vi "ConfigurePigeonMP.vi"(8 "Pigeon Talon":T1, 9 "Pigeon":T6 {"Type" items=["CAN"=352321536, "TalonSRX"=33554432]}, 10 "Right Side":T1, 11 "Left Side":T1) -> (1 "Pigeon":T6 {"Type" items=["CAN"=352321536, "TalonSRX"=33554432]}, 2 "Right Side":T1, 3 "Left Side":T1)   [LabVIEW 2018]
uses:
  <vilib>/Rock Robotics/WPI/ThirdParty/Phoenix-LabVIEW/Pigeon IMU/CTRE_PigeonIMU_DeviceRef.ctl
  <vilib>/Rock Robotics/WPI/ThirdParty/Phoenix-LabVIEW/Pigeon IMU/CTRE_PigeonIMU_ConnectionType.ctl
  <vilib>/Rock Robotics/WPI/MotorControl/WPI_MotorControlDeviceRef.ctl
  <vilib>/Rock Robotics/WPI/MotorControl/WPI_MotorControlType.ctl
  <vilib>/Rock Robotics/SystemInterfaces/DIO/FPGA_DIOPWMChannel.ctl
  <vilib>/Rock Robotics/WPI/PWM/WPI_PWMDeadband.ctl
  <vilib>/Rock Robotics/SystemInterfaces/DIO/FPGA_DIOChannel.ctl
  <vilib>/Rock Robotics/WPI/ThirdParty/Phoenix-LabVIEW/Motor Controller/Controls/CTRE_Phoenix_MotorControl_FeedbackDevice.ctl
  <vilib>/Rock Robotics/WPI/ThirdParty/Phoenix-LabVIEW/Motor Controller/Controls/CTRE_Phoenix_MotorControl_RemoteSourceType.ctl
  <vilib>/Rock Robotics/WPI/ThirdParty/Phoenix-LabVIEW/Motor Controller/Controls/CTRE_Phoenix_MotorControl_SensorTermFeedbackDevice_Enhanced.ctl
  <vilib>/Rock Robotics/WPI/ThirdParty/Phoenix-LabVIEW/Motor Controller/Controls/CTRE_Phoenix_MotorControl_StatusFrameEnhanced.ctl
  <vilib>/Rock Robotics/WPI/ThirdParty/Phoenix-LabVIEW/Motor Controller/Controls/CTRE_Phoenix_MotorControl_NeutralMode.ctl
  <vilib>/Rock Robotics/WPI/ThirdParty/Phoenix-LabVIEW/Motor Controller/Controls/CTRE_Phoenix_MotorControl_ControlMode.ctl
  <vilib>/Rock Robotics/WPI/ThirdParty/Phoenix-LabVIEW/Controls/CTRE_Phoenix_Params.ctl
  <vilib>/Rock Robotics/WPI/ThirdParty/Phoenix-LabVIEW/Motor Controller/Controls/CTRE_Phoenix_MotorControl_ControlFrameEnhanced.ctl
  Constants.vi
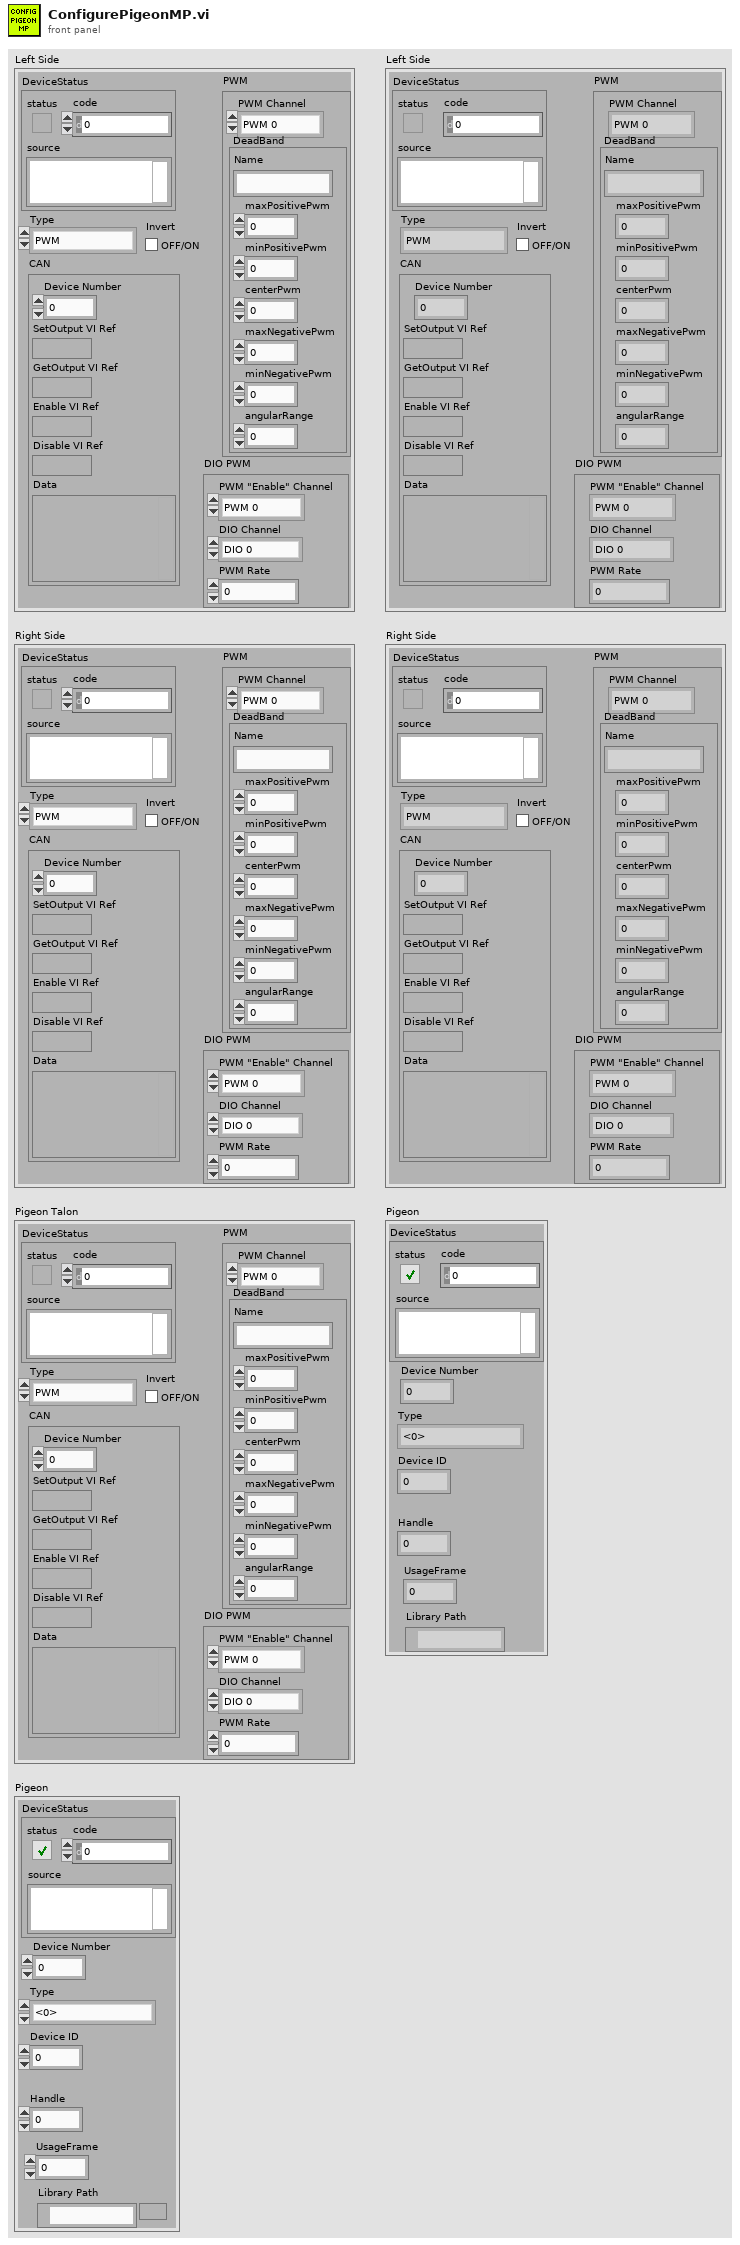
[diagram p1: front panel]
types:
  T1 = typedef "WPI_MotorControlDeviceRef.ctl" = cluster{"DeviceStatus":errorcluster, "Type":T2, "PWM":cluster{"PWM Channel":T3, "DeadBand":T4}, "CAN":cluster{"Device Number":u8, "SetOutput VI Ref":variant, "GetOutput VI Ref":variant, "Enable VI Ref":variant, "Disable VI Ref":variant, "Data":variant}, "Invert":bool, "DIO PWM":cluster{"PWM \"Enable\" Channel":T3, "DIOChannel":T5, "PWM Rate":dbl}}
  T2 = typedef "WPI_MotorControlType.ctl" = enum16{"PWM", "CAN", "DIO PWM"}
  T3 = typedef "FPGA_DIOPWMChannel.ctl" = enum8{"PWM 0", "PWM 1", "PWM 2", "PWM 3", "PWM 4", "PWM 5", "PWM 6", "PWM 7", "PWM 8", "PWM 9", "PWM MXP 0", "PWM MXP 1", "PWM MXP 2", "PWM MXP 3", "PWM MXP 4", "PWM MXP 5", "PWM MXP 6", "PWM MXP 7", "PWM MXP 8", "PWM MXP 9", "Invalid"}
  T4 = typedef "WPI_PWMDeadband.ctl" = cluster{"Name":string, "maxPositivePwm":i32, "minPositivePwm":i32, "centerPwm":i32, "maxNegativePwm":i32, "minNegativePwm":i32, "angularRange":u16}
  T5 = typedef "FPGA_DIOChannel.ctl" = enum8{"DIO 0", "DIO 1", "DIO 2", "DIO 3", "DIO 4", "DIO 5", "DIO 6", "DIO 7", "DIO 8", "DIO 9", "DIO MXP 0", "DIO MXP 1", "DIO MXP 2", "DIO MXP 3", "DIO MXP 4", "DIO MXP 5", "DIO MXP 6", "DIO MXP 7", "DIO MXP 8", "DIO MXP 9", "DIO MXP 10", "DIO MXP 11", "DIO MXP 12", "DIO MXP 13", "DIO MXP 14", "DIO MXP 15", "SPI Port CS1", "SPI Port CS2", "SPI Port CS3", "SPI Port MISO", "SPI Port MOSI", "Invalid"}
  T6 = typedef "CTRE_PigeonIMU_DeviceRef.ctl" = cluster{"DeviceStatus":errorcluster, "Device Number":u8, "Type":T7, "Device ID":u32, "Handle":u64, "UsageFrame":u32, "Library Path":path}
  T7 = typedef "CTRE_PigeonIMU_ConnectionType.ctl" = u32
  T8 = typedef "CTRE_Phoenix_MotorControl_ControlFrameEnhanced.ctl" = u32
  T9 = typedef "CTRE_Phoenix_MotorControl_StatusFrameEnhanced.ctl" = u16
  T10 = typedef "CTRE_Phoenix_Params.ctl" = u16
  T11 = typedef "CTRE_Phoenix_MotorControl_ControlMode.ctl" = u16
  T12 = typedef "CTRE_Phoenix_MotorControl_NeutralMode.ctl" = enum8{"EEPROMSetting", "Override to Coast", "Override to Brake"}
  T13 = typedef "CTRE_Phoenix_MotorControl_FeedbackDevice.ctl" = i8
  T14 = typedef "CTRE_Phoenix_MotorControl_SensorTermFeedbackDevice_Enhanced.ctl" = i8
  T15 = typedef "CTRE_Phoenix_MotorControl_RemoteSourceType.ctl" = enum16{"Off", "Talon SRX Selected Sensor", "Pigeon IMU Yaw", "Pigeon IMU Pitch", "Pigeon IMU Roll", "CANifier Quadrature", "CANifier PWM Input 0", "CANifier PWM Input 1", "CANifier PWM Input 2", "CANifier PWM Input 3", "Gadgeteer Pigeon Yaw", "Gadgeteer Pigeon Pitch", "Gadgeteer Pigeon Roll"}
  T16 = cluster{"kP":dbl, "kI ":dbl, "kD":dbl, "kF":dbl, "I Zone":dbl, "Peak Out":dbl}
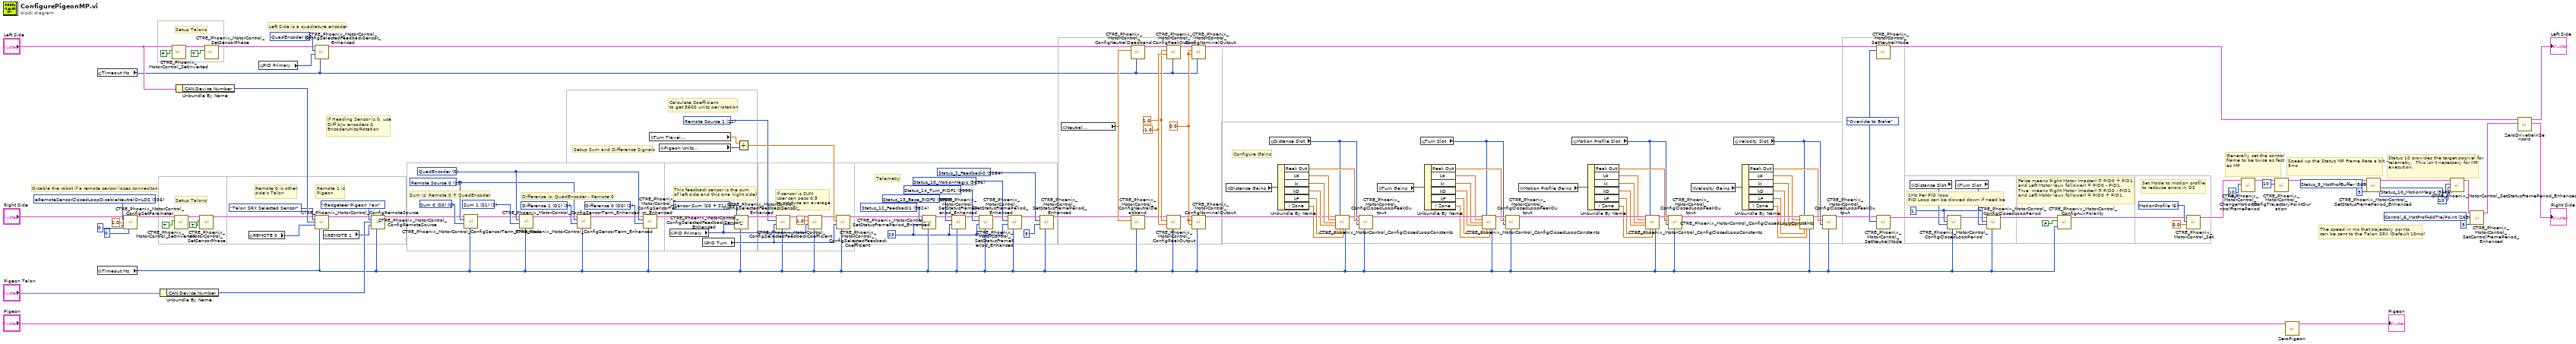
[diagram p0: block diagram]
diagram:
  w6 = T8 262464 items=["Control_3_General"=262272, "Control_4_Advanced"=262336, "Control_5_FeedbackOutputOverride"=262400, "Control_6_MotProfAddTrajPoint"=262464] ("Control Frame")
  w12 = T9 5696 items=["Status_1_General"=5120, "Status_2_Feedback0"=5184, "Status_3_Quadrature"=5248, "Status_4_AinTempVbat"=5312, "Status_6_Misc"=5440, "Status_7_CommStatus"=5504, "Status_8_PulseWidth"=5568, "Status_9_MotProfBuffer"=5632, "Status_10_MotionMagic"=5696, "Status_11_UartGadgeteer"=5760, "Status_12_Feedback1"=5824, "Status_13_Base_PIDF0"=5888, "Status_14_Turn_PIDF1"=5952, "Status_15_FirmwareApiStatus"=6016] ("Status Frame")
  w14 = T9 5632 items=["Status_1_General"=5120, "Status_2_Feedback0"=5184, "Status_3_Quadrature"=5248, "Status_4_AinTempVbat"=5312, "Status_6_Misc"=5440, "Status_7_CommStatus"=5504, "Status_8_PulseWidth"=5568, "Status_9_MotProfBuffer"=5632, "Status_10_MotionMagic"=5696, "Status_11_UartGadgeteer"=5760, "Status_12_Feedback1"=5824, "Status_13_Base_PIDF0"=5888, "Status_14_Turn_PIDF1"=5952, "Status_15_FirmwareApiStatus"=6016] ("Status Frame")
  w20 = T10 336 items=["eOnBoot_BrakeMode"=31, "eQuadFilterEn"=91, "eQuadIdxPolarity"=108, "eClearPositionOnIdx"=100, "eMotionProfileHasUnderrunErr"=119, "eMotionProfileTrajectoryPointDurationMs"=120, "eClearPosOnLimitF"=144, "eClearPosOnLimitR"=145, "eStatusFramePeriod"=300, "eOpenLoopRamp"=301, "eClosedLoopRamp"=302, "eNeutralDeadband"=303, "ePeakPosOutput"=305, "eNominalPosOutput"=306, "ePeakNegOutput"=307, "eNominalNegOutput"=308, "eProfileParamSlot_P"=310, "eProfileParamSlot_I"=311, "eProfileParamSlot_D"=312, "eProfileParamSlot_F"=313, "eProfileParamSlot_IZone"=314, "eProfileParamSlot_AllowableErr"=315, "eProfileParamSlot_MaxIAccum"=316, "eClearPositionOnLimitF"=320, "eClearPositionOnLimitR"=321, "eClearPositionOnQuadIdx"=322, "eSampleVelocityPeriod"=325, "eSampleVelocityWindow"=326, "eFeedbackSensorType"=330, "eSelectedSensorPosition"=331, "eFeedbackNotContinuous"=332, "eRemoteSensorSource"=333, "eRemoteSensorDeviceID"=334, "eSensorTerm"=335, "eRemoteSensorClosedLoopDisableNeutralOnLOS"=336, "eForwardSoftLimitThreshold"=340, "eReverseSoftLimitThreshold"=341, "eForwardSoftLimitEnable"=342, "eReverseSoftLimitEnable"=343, "eNominalBatteryVoltage"=350, "eBatterVoltageFilterSize"=351, "eContinuousCurrentLimitAmps"=360, "eContinuousCurrentLimitMs"=361, "ePeakCurrentLimitAmps"=362, "eClosedLoopIAccum"=370, "eCustomParam"=380, "eStickyFaults"=390, "eAnalogPosition"=400, "eQuadraturePosition"=401, "ePulseWidthPosition"=402, "eMotMag_Accel"=410, "eMotMag_VelCruise"=411, "eLimitSwitchSource"=421, "eLimitSwitchNormClosedAndDis"=422, "eLimitSwitchDisabledNeutralOnLOS"=423, "eLimitSwitchRemoteDevID"=424] ("Parameter")
  w32 = T11 6 items=["PercentOutput"=0, "Position"=1, "Velocity"=2, "Current"=3, "Follower"=5, "MotionProfile"=6, "MotionMagic"=7, "MotionProfileArc"=10, "Disabled"=15] ("Control Mode")
  w140 = 1 ("loopTimeMs")
  w136 = CTRE_Phoenix_MotorControl_NeutralMode."Override to Brake" ("Motor Control Neutral Mode")
  w97 = 0.0 ("Forward Nominal Percent Output")
  w94 = -1.0 ("Reverse Peak Percent Output")
  w93 = 1.0 ("Forward Peak Percent Output")
  w29 = 20 ("periodMs")
  w86 = T9 5184 items=["Status_1_General"=5120, "Status_2_Feedback0"=5184, "Status_3_Quadrature"=5248, "Status_4_AinTempVbat"=5312, "Status_6_Misc"=5440, "Status_7_CommStatus"=5504, "Status_8_PulseWidth"=5568, "Status_9_MotProfBuffer"=5632, "Status_10_MotionMagic"=5696, "Status_11_UartGadgeteer"=5760, "Status_12_Feedback1"=5824, "Status_13_Base_PIDF0"=5888, "Status_14_Turn_PIDF1"=5952, "Status_15_FirmwareApiStatus"=6016] ("Status Frame")
  w85 = T9 5696 items=["Status_1_General"=5120, "Status_2_Feedback0"=5184, "Status_3_Quadrature"=5248, "Status_4_AinTempVbat"=5312, "Status_6_Misc"=5440, "Status_7_CommStatus"=5504, "Status_8_PulseWidth"=5568, "Status_9_MotProfBuffer"=5632, "Status_10_MotionMagic"=5696, "Status_11_UartGadgeteer"=5760, "Status_12_Feedback1"=5824, "Status_13_Base_PIDF0"=5888, "Status_14_Turn_PIDF1"=5952, "Status_15_FirmwareApiStatus"=6016] ("Status Frame")
  w84 = T9 5952 items=["Status_1_General"=5120, "Status_2_Feedback0"=5184, "Status_3_Quadrature"=5248, "Status_4_AinTempVbat"=5312, "Status_6_Misc"=5440, "Status_7_CommStatus"=5504, "Status_8_PulseWidth"=5568, "Status_9_MotProfBuffer"=5632, "Status_10_MotionMagic"=5696, "Status_11_UartGadgeteer"=5760, "Status_12_Feedback1"=5824, "Status_13_Base_PIDF0"=5888, "Status_14_Turn_PIDF1"=5952, "Status_15_FirmwareApiStatus"=6016] ("Status Frame")
  w83 = T9 5888 items=["Status_1_General"=5120, "Status_2_Feedback0"=5184, "Status_3_Quadrature"=5248, "Status_4_AinTempVbat"=5312, "Status_6_Misc"=5440, "Status_7_CommStatus"=5504, "Status_8_PulseWidth"=5568, "Status_9_MotProfBuffer"=5632, "Status_10_MotionMagic"=5696, "Status_11_UartGadgeteer"=5760, "Status_12_Feedback1"=5824, "Status_13_Base_PIDF0"=5888, "Status_14_Turn_PIDF1"=5952, "Status_15_FirmwareApiStatus"=6016] ("Status Frame")
  w82 = T9 5824 items=["Status_1_General"=5120, "Status_2_Feedback0"=5184, "Status_3_Quadrature"=5248, "Status_4_AinTempVbat"=5312, "Status_6_Misc"=5440, "Status_7_CommStatus"=5504, "Status_8_PulseWidth"=5568, "Status_9_MotProfBuffer"=5632, "Status_10_MotionMagic"=5696, "Status_11_UartGadgeteer"=5760, "Status_12_Feedback1"=5824, "Status_13_Base_PIDF0"=5888, "Status_14_Turn_PIDF1"=5952, "Status_15_FirmwareApiStatus"=6016] ("Status Frame")
  w27 = T13 12 items=["None"=-1, "QuadEncoder"=0, "Analog"=2, "Tachometer"=4, "Pulse Width Encoded Position"=8, "Sensor Sum (S0 + S1)"=9, "Sensor Difference (D0 - D1)"=10, "Remote Source 0"=11, "Remote Source 1"=12, "Software Emulated"=15] ("Feedback Device")
  w69 = T13 9 items=["None"=-1, "QuadEncoder"=0, "Analog"=2, "Tachometer"=4, "Pulse Width Encoded Position"=8, "Sensor Sum (S0 + S1)"=9, "Sensor Difference (D0 - D1)"=10, "Remote Source 0"=11, "Remote Source 1"=12, "Software Emulated"=15] ("Feedback Device")
  w67 = u16 2 items=["Sum 0 (S0)", "Sum 1 (S1)", "Difference 0 (D0)", "Difference 1 (D1)"] ("Sensor Term")
  w66 = u16 3 items=["Sum 0 (S0)", "Sum 1 (S1)", "Difference 0 (D0)", "Difference 1 (D1)"] ("Sensor Term")
  w61 = u16 1 items=["Sum 0 (S0)", "Sum 1 (S1)", "Difference 0 (D0)", "Difference 1 (D1)"] ("Sensor Term")
  w65 = T14 0 items=["None"=-1, "QuadEncoder"=0, "Analog"=2, "Tachometer"=4, "Pulse Width Encoded Position"=8, "Remote Source 0"=11, "Remote Source 1"=12, "Software Emulated"=15] ("Feedback Device")
  w59 = u16 0 items=["Sum 0 (S0)", "Sum 1 (S1)", "Difference 0 (D0)", "Difference 1 (D1)"] ("Sensor Term")
  w64 = T14 11 items=["None"=-1, "QuadEncoder"=0, "Analog"=2, "Tachometer"=4, "Pulse Width Encoded Position"=8, "Remote Source 0"=11, "Remote Source 1"=12, "Software Emulated"=15] ("Feedback Device")
  w47 = T13 0 items=["None"=-1, "QuadEncoder"=0, "Analog"=2, "Tachometer"=4, "Pulse Width Encoded Position"=8, "Sensor Sum (S0 + S1)"=9, "Sensor Difference (D0 - D1)"=10, "Remote Source 0"=11, "Remote Source 1"=12, "Software Emulated"=15] ("Feedback Device")
  # "The speed in ms that trajectory points\ncan be sent to the Talon SRX (Default 10ms)"
  # "Generally set the control frame to be twice as fast as MP"
  # "Status 10 provides the target pos/vel for telemetry.  This isn't necessary for MP execution."
  # "Speed up the Status MP Frame Rate a bit - 5ms"
  # "Disable the robot if a remote sensor loses conneciton"
  # "Set Mode to motion profile\nto redsuce errors in DS"
  # "False means Right Motor (master) = PID0 + PID1, \nand Left Motor (aux follower) = PID0 - PID1.\nTrue  means Right Motor (master) = PID0 - PID1, \nand Left Motor (aux follower) = PID0 + PID1."
  # "1Ms Per PID loop\nPID Loop can be slowed down if need be"
  # "Configure Gains"
  # "Setup Talons"
  # "Telemetry"
  # "If sensor is SUM,\nUser can pass 0.5\nto produce an average"
  # "Calculate Coefficient\nto get 3600 units per rotation"
  # "If Heading Sensor is 0, use \nDiff b/w encoders &\nEncoderUnits/Rotation"
  # "This feedback sensor is the sum\nof left side and this one (right side)"
  # "Difference is: QuadEncoder - Remote 0"
  # "Sum is: Remote 0 + QuadEncoder"
  # "Setup Sum and Difference Signals"
  # "Remote 1 is\nPigeon"
  # "Remote 0 is other\nside's Talon"
  # "Left Side is a quadrature encoder"
  # "Setup Talons"
  n1 = global read "Constants.vi" "Timeout Ms"() -> (w26:i32)
  n2 = global read "Constants.vi" "Timeout Ms"() -> (w38:i32)
  n3 = call <vilib>:"CTRE_Phoenix_MotorControl_ConfigSetParameter.vi"("PhoenixMotorControlDevRef"="Right Side", "Parameter"=w20, "value"=1.0, "subValue"=u8 0, "ordinal"=0) -> ("PhoenixMotorControlDevRef"=w15:T1)  [unwired: 9 in, 1 out]
  n4 = Unbundle By Name("Pigeon Talon") -> ("CAN.Device Number"=w56:u8)
  n5 = call <vilib>:"CTRE_Phoenix_MotorControl_SetInverted.vi"("Invert?"=FALSE, "PhoenixMotorControlDevRef"="Left Side") -> ("PhoenixMotorControlDevRef"=w42:T1)  [unwired: 8 in, 1 out]
  n6 = call <vilib>:"CTRE_Phoenix_MotorControl_SetInverted.vi"("Invert?"=TRUE, "PhoenixMotorControlDevRef"=w15) -> ("PhoenixMotorControlDevRef"=w43:T1)  [unwired: 8 in, 1 out]
  n7 = Unbundle By Name("Left Side") -> ("CAN.Device Number"=w51:u8)
  n8 = call <vilib>:"CTRE_Phoenix_MotorControl_SetSensorPhase.vi"("PhaseSensor"=TRUE, "PhoenixMotorControlDevRef"=w43) -> ("PhoenixMotorControlDevRef"=w48:T1)  [unwired: 8 in, 1 out]
  n9 = call <vilib>:"CTRE_Phoenix_MotorControl_SetSensorPhase.vi"("PhaseSensor"=TRUE, "PhoenixMotorControlDevRef"=w42) -> ("PhoenixMotorControlDevRef"=w46:T1)  [unwired: 8 in, 1 out]
  n10 = global read "Constants.vi" "REMOTE 0"() -> (w52:i32)
  n11 = global read "Constants.vi" "PID Primary"() -> (w143:i32)
  n12 = call <vilib>:"CTRE_Phoenix_MotorControl_ConfigSelectedFeedbackSensor_Enhanced.vi"("timeoutMs"=w26, "pidLoopIdx"=w143, "Feedback Device"=w47, "PhoenixMotorControlDevRef"=w46) -> ("PhoenixMotorControlDevRef"=w90:T1)  [unwired: 6 in, 1 out]
  n13 = call <vilib>:"CTRE_Phoenix_MotorControl_ConfigRemoteSource.vi"("PhoenixMotorControlDevRef"=w48, "Remote Device Type"=CTRE_Phoenix_MotorControl_RemoteSourceType."Talon SRX Selected Sensor", "Remote Device ID"=w51, "Source Index (0/1)"=w52, "timeoutMs"=w38) -> ("PhoenixMotorControlDevRef"=w53:T1)  [unwired: 9 in, 1 out]
  n14 = global read "Constants.vi" "REMOTE 1"() -> (w57:i32)
  n15 = call <vilib>:"CTRE_Phoenix_MotorControl_ConfigRemoteSource.vi"("PhoenixMotorControlDevRef"=w53, "Remote Device Type"=CTRE_Phoenix_MotorControl_RemoteSourceType."Gadgeteer Pigeon Yaw", "Remote Device ID"=w56, "Source Index (0/1)"=w57, "timeoutMs"=w38) -> ("PhoenixMotorControlDevRef"=w58:T1)  [unwired: 9 in, 1 out]
  n16 = call <vilib>:"CTRE_Phoenix_MotorControl_ConfigSensorTerm_Enhanced.vi"("timeoutMs"=w38, "Sensor Term"=w59, "Feedback Device"=w64, "PhoenixMotorControlDevRef"=w58) -> ("PhoenixMotorControlDevRef"=w60:T1)  [unwired: 6 in, 1 out]
  n17 = call <vilib>:"CTRE_Phoenix_MotorControl_ConfigSensorTerm_Enhanced.vi"("timeoutMs"=w38, "Sensor Term"=w61, "Feedback Device"=w65, "PhoenixMotorControlDevRef"=w60) -> ("PhoenixMotorControlDevRef"=w63:T1)  [unwired: 6 in, 1 out]
  n18 = call <vilib>:"CTRE_Phoenix_MotorControl_ConfigSensorTerm_Enhanced.vi"("timeoutMs"=w38, "Sensor Term"=w66, "Feedback Device"=w64, "PhoenixMotorControlDevRef"=w63) -> ("PhoenixMotorControlDevRef"=w62:T1)  [unwired: 6 in, 1 out]
  n19 = call <vilib>:"CTRE_Phoenix_MotorControl_ConfigSensorTerm_Enhanced.vi"("timeoutMs"=w38, "Sensor Term"=w67, "Feedback Device"=w65, "PhoenixMotorControlDevRef"=w62) -> ("PhoenixMotorControlDevRef"=w68:T1)  [unwired: 6 in, 1 out]
  n20 = global read "Constants.vi" "Turn Travel\nUnits Per Rotation"() -> (w75:dbl)
  n21 = global read "Constants.vi" "Pigeon Units\nPer Rotatoin"() -> (w28:i32)
  n22 = global read "Constants.vi" "PID Primary"() -> (w142:i32)
  n23 = global read "Constants.vi" "PID Turn"() -> (w74:i32)
  n24 = call <vilib>:"CTRE_Phoenix_MotorControl_ConfigSelectedFeedbackSensor_Enhanced.vi"("timeoutMs"=w38, "pidLoopIdx"=w142, "Feedback Device"=w69, "PhoenixMotorControlDevRef"=w68) -> ("PhoenixMotorControlDevRef"=w70:T1)  [unwired: 6 in, 1 out]
  n25 = Divide(x=w75, y=w28) -> (x/y=w76:dbl)
  n26 = call <vilib>:"CTRE_Phoenix_MotorControl_ConfigSelectedFeedbackSensor_Enhanced.vi"("timeoutMs"=w38, "pidLoopIdx"=w74, "Feedback Device"=w27, "PhoenixMotorControlDevRef"=w70) -> ("PhoenixMotorControlDevRef"=w71:T1)  [unwired: 6 in, 1 out]
  n27 = call <vilib>:"CTRE_Phoenix_MotorControl_ConfigSelectedFeedbackCoefficient.vi"("timoutMs"=w38, "pidIdx"=w142, "coefficient"=1.0, "PhoenixMotorControlDevRef"=w71) -> ("PhoenixMotorControlDevRef"=w73:T1)  [unwired: 6 in, 1 out]
  n28 = call <vilib>:"CTRE_Phoenix_MotorControl_ConfigSelectedFeedbackCoefficient.vi"("timoutMs"=w38, "pidIdx"=w74, "coefficient"=w76, "PhoenixMotorControlDevRef"=w73) -> ("PhoenixMotorControlDevRef"=w77:T1)  [unwired: 6 in, 1 out]
  n29 = call <vilib>:"CTRE_Phoenix_MotorControl_SetStatusFramePeriod_Enhanced.vi"("timeoutMs"=w38, "periodMs"=w29, "Status Frame"=w82, "PhoenixMotorControlDevRef"=w77) -> ("PhoenixMotorControlDevRef"=w78:T1)  [unwired: 6 in, 1 out]
  n30 = call <vilib>:"CTRE_Phoenix_MotorControl_SetStatusFramePeriod_Enhanced.vi"("timeoutMs"=w38, "periodMs"=w29, "Status Frame"=w83, "PhoenixMotorControlDevRef"=w78) -> ("PhoenixMotorControlDevRef"=w79:T1)  [unwired: 6 in, 1 out]
  n31 = call <vilib>:"CTRE_Phoenix_MotorControl_SetStatusFramePeriod_Enhanced.vi"("timeoutMs"=w38, "periodMs"=w29, "Status Frame"=w84, "PhoenixMotorControlDevRef"=w79) -> ("PhoenixMotorControlDevRef"=w80:T1)  [unwired: 6 in, 1 out]
  n32 = call <vilib>:"CTRE_Phoenix_MotorControl_SetStatusFramePeriod_Enhanced.vi"("timeoutMs"=w38, "periodMs"=w29, "Status Frame"=w85, "PhoenixMotorControlDevRef"=w80) -> ("PhoenixMotorControlDevRef"=w81:T1)  [unwired: 6 in, 1 out]
  n33 = call <vilib>:"CTRE_Phoenix_MotorControl_SetStatusFramePeriod_Enhanced.vi"("timeoutMs"=w38, "periodMs"=5, "Status Frame"=w86, "PhoenixMotorControlDevRef"=w81) -> ("PhoenixMotorControlDevRef"=w88:T1)  [unwired: 6 in, 1 out]
  n34 = global read "Constants.vi" "Neutral\nDeadband"() -> (w91:dbl)
  n35 = call <vilib>:"CTRE_Phoenix_MotorControl_ConfigNeutralDeadband.vi"("timeoutMs"=w26, "Percent Deadband"=w91, "PhoenixMotorControlDevRef"=w90) -> ("PhoenixMotorControlDevRef"=w92:T1)  [unwired: 7 in, 1 out]
  n36 = call <vilib>:"CTRE_Phoenix_MotorControl_ConfigNeutralDeadband.vi"("timeoutMs"=w38, "Percent Deadband"=w91, "PhoenixMotorControlDevRef"=w88) -> ("PhoenixMotorControlDevRef"=w89:T1)  [unwired: 7 in, 1 out]
  n37 = call <vilib>:"CTRE_Phoenix_MotorControl_ConfigPeakOutput.vi"("timeoutMs"=w26, "Reverse Peak Percent Output"=w94, "Forward Peak Percent Output"=w93, "PhoenixMotorControlDevRef"=w92) -> ("PhoenixMotorControlDevRef"=w96:T1)  [unwired: 6 in, 1 out]
  n38 = call <vilib>:"CTRE_Phoenix_MotorControl_ConfigPeakOutput.vi"("timeoutMs"=w38, "Reverse Peak Percent Output"=w94, "Forward Peak Percent Output"=w93, "PhoenixMotorControlDevRef"=w89) -> ("PhoenixMotorControlDevRef"=w95:T1)  [unwired: 6 in, 1 out]
  n39 = call <vilib>:"CTRE_Phoenix_MotorControl_ConfigNominalOutput.vi"("timeoutMs"=w26, "Reverse Nominal Percent Output"=w97, "Forward Nominal Percent Output"=w97, "PhoenixMotorControlDevRef"=w96) -> ("PhoenixMotorControlDevRef"=w135:T1)  [unwired: 6 in, 1 out]
  n40 = call <vilib>:"CTRE_Phoenix_MotorControl_ConfigNominalOutput.vi"("timeoutMs"=w38, "Reverse Nominal Percent Output"=w97, "Forward Nominal Percent Output"=w97, "PhoenixMotorControlDevRef"=w95) -> ("PhoenixMotorControlDevRef"=w98:T1)  [unwired: 6 in, 1 out]
  n41 = global read "Constants.vi" "Distance Gains"() -> (w99:T16)
  n42 = global read "Constants.vi" "Distance Slot"() -> (w35:i32)
  n43 = Unbundle By Name(w99) -> ("Peak Out"=w106:dbl, "kP"=w100:dbl, "kI"=w101:dbl, "kD"=w102:dbl, "kF"=w103:dbl, "I Zone"=w104:dbl)
  n44 = call <vilib>:"CTRE_Phoenix_MotorControl_ConfigClosedLoopConstants.vi"("PhoenixMotorControlDevRef"=w98, "slotIdx"=w35, "P"=w100, "I"=w101, "D"=w102, "F"=w103, "I Zone"=w104, "timeoutMs"=w38) -> ("PhoenixMotorControlDevRef"=w105:T1)  [unwired: 6 in, 1 out]
  n45 = call <vilib>:"CTRE_Phoenix_MotorControl_ConfigClosedLoopPeakOutput.vi"("timoutMs"=w38, "slotIdx"=w35, "peakOutput"=w106, "PhoenixMotorControlDevRef"=w105) -> ("PhoenixMotorControlDevRef"=w131:T1)  [unwired: 6 in, 1 out]
  n46 = global read "Constants.vi" "Turn Gains"() -> (w114:T16)
  n47 = global read "Constants.vi" "Turn Slot"() -> (w34:i32)
  n48 = Unbundle By Name(w114) -> ("Peak Out"=w107:dbl, "kP"=w113:dbl, "kI"=w112:dbl, "kD"=w111:dbl, "kF"=w110:dbl, "I Zone"=w109:dbl)
  n49 = call <vilib>:"CTRE_Phoenix_MotorControl_ConfigClosedLoopConstants.vi"("PhoenixMotorControlDevRef"=w131, "slotIdx"=w34, "P"=w113, "I"=w112, "D"=w111, "F"=w110, "I Zone"=w109, "timeoutMs"=w38) -> ("PhoenixMotorControlDevRef"=w108:T1)  [unwired: 6 in, 1 out]
  n50 = call <vilib>:"CTRE_Phoenix_MotorControl_ConfigClosedLoopPeakOutput.vi"("timoutMs"=w38, "slotIdx"=w34, "peakOutput"=w107, "PhoenixMotorControlDevRef"=w108) -> ("PhoenixMotorControlDevRef"=w132:T1)  [unwired: 6 in, 1 out]
  n51 = global read "Constants.vi" "Motion Profile Gains"() -> (w115:T16)
  n52 = global read "Constants.vi" "Motion Profile Slot"() -> (w36:i32)
  n53 = Unbundle By Name(w115) -> ("Peak Out"=w122:dbl, "kP"=w116:dbl, "kI"=w117:dbl, "kD"=w118:dbl, "kF"=w119:dbl, "I Zone"=w120:dbl)
  n54 = call <vilib>:"CTRE_Phoenix_MotorControl_ConfigClosedLoopConstants.vi"("PhoenixMotorControlDevRef"=w132, "slotIdx"=w36, "P"=w116, "I"=w117, "D"=w118, "F"=w119, "I Zone"=w120, "timeoutMs"=w38) -> ("PhoenixMotorControlDevRef"=w121:T1)  [unwired: 6 in, 1 out]
  n55 = call <vilib>:"CTRE_Phoenix_MotorControl_ConfigClosedLoopPeakOutput.vi"("timoutMs"=w38, "slotIdx"=w36, "peakOutput"=w122, "PhoenixMotorControlDevRef"=w121) -> ("PhoenixMotorControlDevRef"=w133:T1)  [unwired: 6 in, 1 out]
  n56 = global read "Constants.vi" "Velocity Gains"() -> (w130:T16)
  n57 = global read "Constants.vi" "Velocity Slot"() -> (w33:i32)
  n58 = Unbundle By Name(w130) -> ("Peak Out"=w123:dbl, "kP"=w129:dbl, "kI"=w128:dbl, "kD"=w127:dbl, "kF"=w126:dbl, "I Zone"=w125:dbl)
  n59 = call <vilib>:"CTRE_Phoenix_MotorControl_ConfigClosedLoopConstants.vi"("PhoenixMotorControlDevRef"=w133, "slotIdx"=w33, "P"=w129, "I"=w128, "D"=w127, "F"=w126, "I Zone"=w125, "timeoutMs"=w38) -> ("PhoenixMotorControlDevRef"=w124:T1)  [unwired: 6 in, 1 out]
  n60 = call <vilib>:"CTRE_Phoenix_MotorControl_ConfigClosedLoopPeakOutput.vi"("timoutMs"=w38, "slotIdx"=w33, "peakOutput"=w123, "PhoenixMotorControlDevRef"=w124) -> ("PhoenixMotorControlDevRef"=w134:T1)  [unwired: 6 in, 1 out]
  n61 = call <vilib>:"CTRE_Phoenix_MotorControl_SetNeutralMode.vi"("Motor Control Neutral Mode"=w136, "PhoenixMotorControlDevRef"=w135) -> ("PhoenixMotorControlDevRef"=w23:T1)  [unwired: 8 in, 1 out]
  n62 = call <vilib>:"CTRE_Phoenix_MotorControl_SetNeutralMode.vi"("Motor Control Neutral Mode"=w136, "PhoenixMotorControlDevRef"=w134) -> ("PhoenixMotorControlDevRef"=w137:T1)  [unwired: 8 in, 1 out]
  n63 = global read "Constants.vi" "Distance Slot"() -> (w138:i32)
  n64 = call <vilib>:"CTRE_Phoenix_MotorControl_ConfigClosedLoopPeriod.vi"("timoutMs"=w38, "slotIdx"=w138, "loopTimeMs"=w140, "PhoenixMotorControlDevRef"=w137) -> ("PhoenixMotorControlDevRef"=w139:T1)  [unwired: 6 in, 1 out]
  n65 = global read "Constants.vi" "Turn Slot"() -> (w141:i32)
  n66 = call <vilib>:"CTRE_Phoenix_MotorControl_ConfigClosedLoopPeriod.vi"("timoutMs"=w38, "slotIdx"=w141, "loopTimeMs"=w140, "PhoenixMotorControlDevRef"=w139) -> ("PhoenixMotorControlDevRef"=w39:T1)  [unwired: 6 in, 1 out]
  n67 = call <vilib>:"CTRE_Phoenix_MotorControl_ConfigAuxPolarity.vi"("timeoutMs"=w38, "Invert"=FALSE, "PhoenixMotorControlDevRef"=w39) -> ("PhoenixMotorControlDevRef"=w30:T1)  [unwired: 7 in, 1 out]
  n68 = call <vilib>:"CTRE_Phoenix_MotorControl_Set.vi"("Output"=0.0, "Control Mode"=w32, "PhoenixMotorControlDevRef"=w30) -> ("PhoenixMotorControlDevRef"=w3:T1)  [unwired: 7 in, 1 out]
  n69 = call <vilib>:"CTRE_Phoenix_MotorControl_ChangeMotionControlFramePeriod.vi"("periodMs"=10, "PhoenixMotorControlDevRef"=w3) -> ("PhoenixMotorControlDevRef"=w9:T1)  [unwired: 8 in, 1 out]
  n70 = call <vilib>:"CTRE_Phoenix_MotorControl_ConfigTrajectoryPointDuration.vi"("durationMs"=10, "PhoenixMotorControlDevRef"=w9) -> ("PhoenixMotorControlDevRef"=w8:T1)  [unwired: 8 in, 1 out]
  n71 = call "ZeroPigeon.vi"("Pigeon"="Pigeon") -> ("Pigeon"=→"Pigeon":T6)  [unwired: 8 in]
  n72 = call <vilib>:"CTRE_Phoenix_MotorControl_SetStatusFramePeriod_Enhanced.vi"("periodMs"=5, "Status Frame"=w14, "PhoenixMotorControlDevRef"=w8) -> ("PhoenixMotorControlDevRef"=w10:T1)  [unwired: 7 in, 1 out]
  n73 = call <vilib>:"CTRE_Phoenix_MotorControl_SetStatusFramePeriod_Enhanced.vi"("periodMs"=10, "Status Frame"=w12, "PhoenixMotorControlDevRef"=w10) -> ("PhoenixMotorControlDevRef"=w5:T1)  [unwired: 7 in, 1 out]
  n74 = call <vilib>:"CTRE_Phoenix_MotorControl_SetControlFramePeriod_Enhanced.vi"("periodMs"=5, "Control Frame"=w6, "MotorControl Device Ref"=w5) -> ("PhoenixMotorControlDevRef"=w2:T1)  [unwired: 7 in, 1 out]
  n75 = call "ZeroDrivetrainSensors.vi"("Talon 2"=w2, "Talon 1"=w23) -> ("Talon 2"=→"Right Side":T1, "Talon 1"=→"Left Side":T1)  [unwired: 8 in]
